vi "试验舱仿真器传递函数-带自然冷却10ms.vi"() -> ()   [LabVIEW 2018]
panel:
  out "波形图表":cluster{"上限":dbl, "上限":dbl, "上限":dbl}(graph)
  in  "自然冷却按钮":bool
  out "1.8m试验仓仓内温度":dbl(graph)
  out "1.8m试验仓仓内压力":dbl(graph)=-0.0229152
  out "1M8仓温度仿真":dbl(slide)=73.625 scale=0.0..250.0
  out "1M8仓压力仿真":dbl(slide)=-0.0229152 scale=0.0..1.0
  out "压力":dbl
  out "f 5":dbl format="%.3f"
  out "d排气影响压力":dbl
  out "f 4":dbl format="%.3f"
  out "d进蒸汽影响压力":dbl
  out "f 3":dbl format="%.3f"
  out "d进空气影响压力":dbl
  out "f 2":dbl format="%.3f"
  out "d进空气影响温度":dbl
  out "f":dbl format="%.3f"
  out "d进蒸汽影响温度":dbl
  out "温度":dbl
  # "试验舱"
  # "压力"
  # "温度"
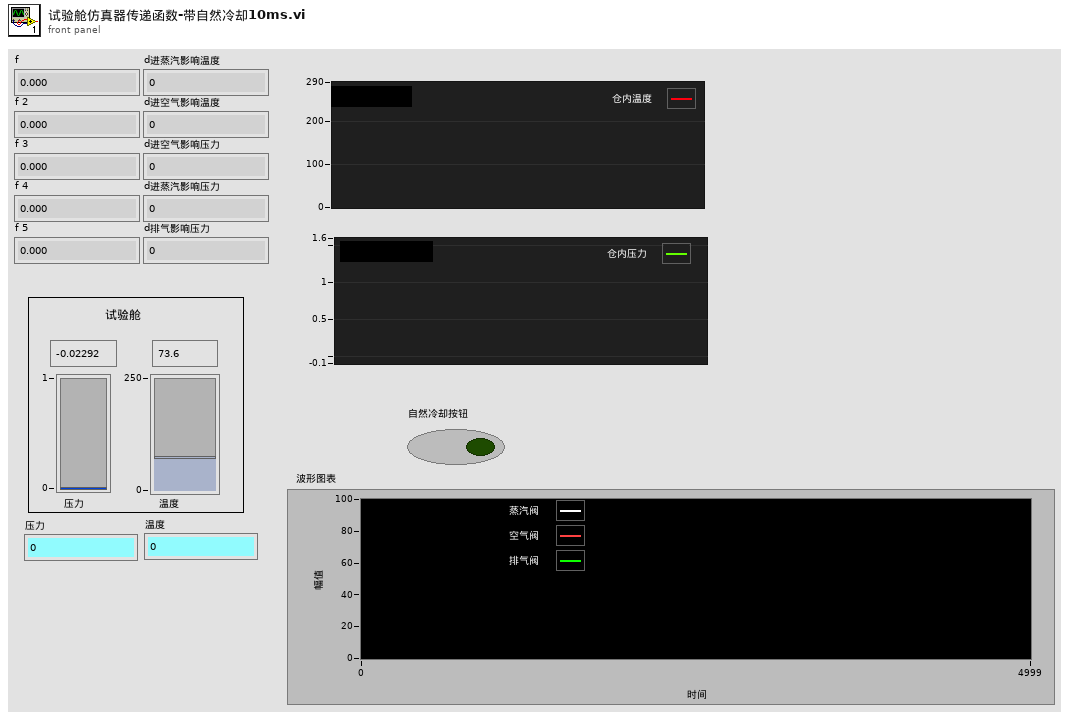
[diagram p1: front panel]
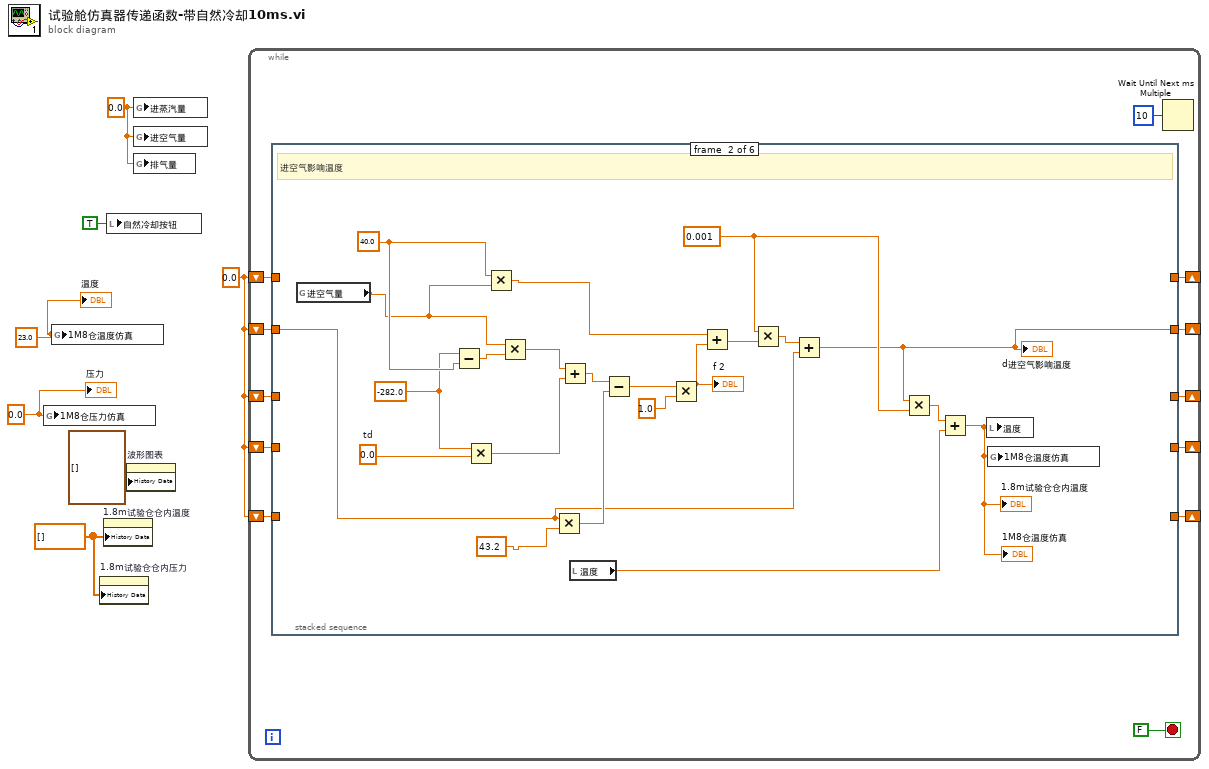
[diagram p0: block diagram]
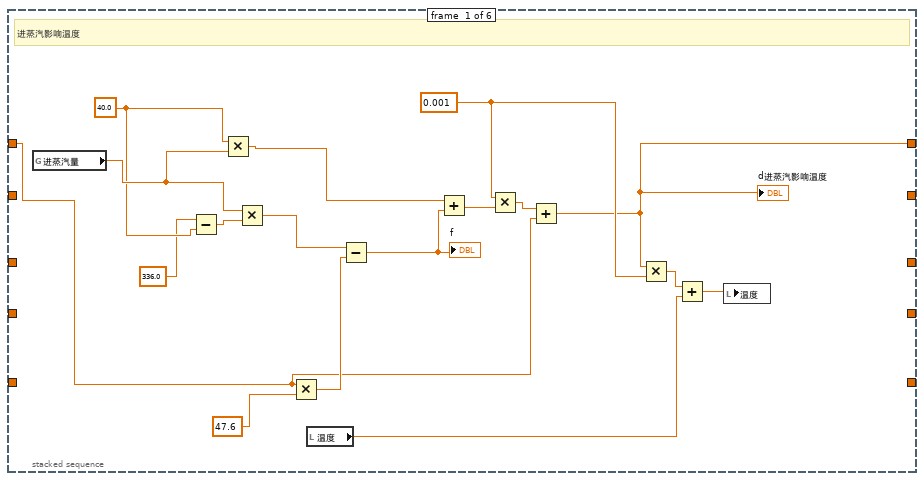
[diagram p2: hidden frame]
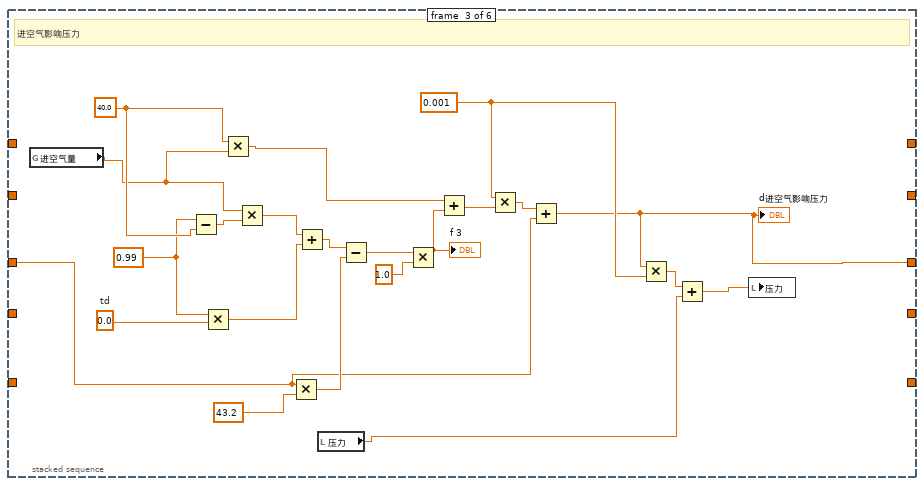
[diagram p3: hidden frame]
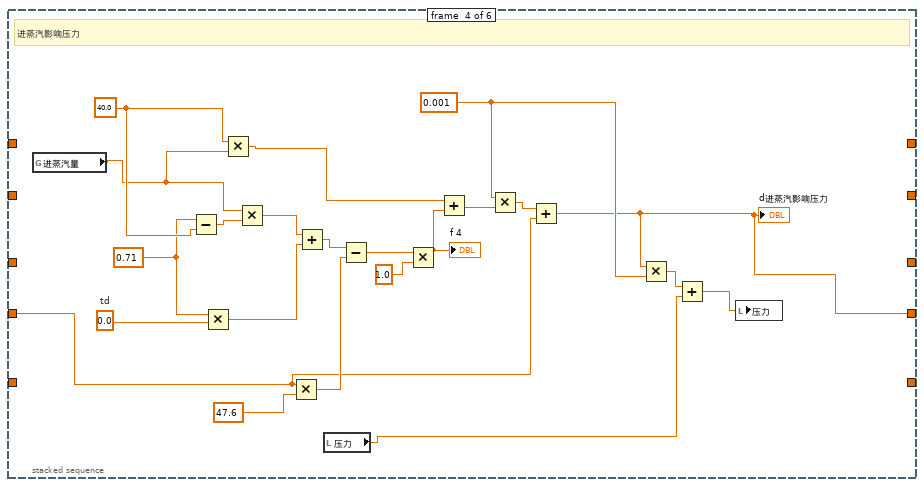
[diagram p4: hidden frame]
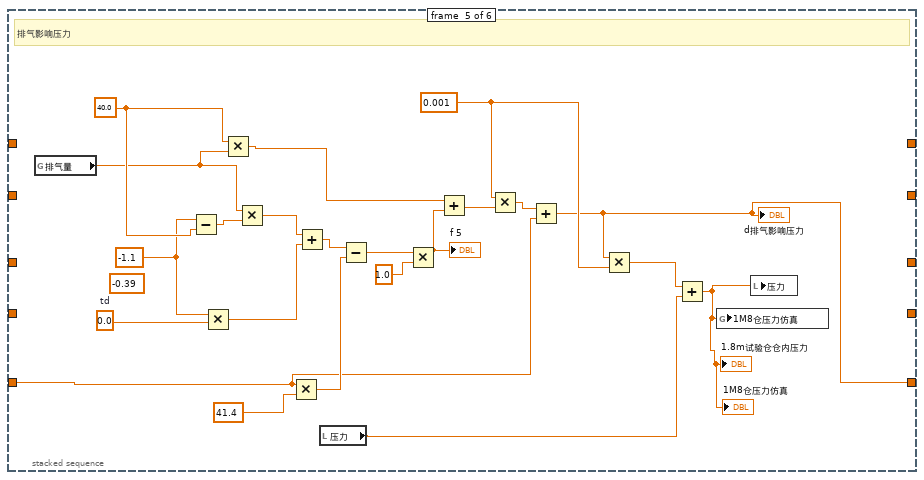
[diagram p5: hidden frame]
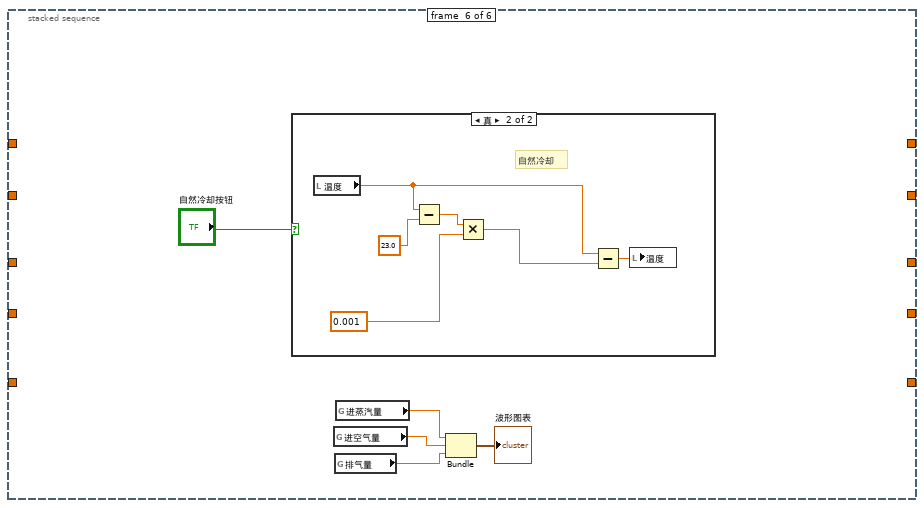
[diagram p6: hidden frame]
diagram:
  w3 = dbl[] [] ("历史数据")
  w6 = 0.0
  w7 = 0.0 ("进蒸汽量")
  w5 = 23.0 ("1.2m试验仓仓内温度")
  w4 = 0.0 ("1m2舱温度峰值")
  n1 = global write "全局变量.vi" "1M8仓压力仿真"(w4) -> ()
  n2 = global write "全局变量.vi" "1M8仓温度仿真"(w5) -> ()
  n3 = property on="1.8m试验仓仓内压力" class="WFChart (严格)"("History Data"=w3) -> ()  [unwired: 2 in, 2 out]
  n4 = property on="1.8m试验仓仓内温度" class="WFChart (严格)"("History Data"=w3) -> ()  [unwired: 2 in, 2 out]
  n5 = local write "自然冷却按钮"(TRUE ("自然冷却按钮")) -> ()
  n6 = property on="波形图表" class="WFChart (严格)"("History Data"=cluster{"上限":dbl, "上限":dbl, "上限":dbl}[] [] ("历史数据")) -> ()  [unwired: 2 in, 2 out]
  n7 = global write "全局变量.vi" "进蒸汽量"(w7) -> ()
  n8 = global write "全局变量.vi" "进空气量"(w7) -> ()
  n9 = global write "全局变量.vi" "排气量"(w7) -> ()
  n10 = while {
    shift-right: [w16] -> _
    shift-left: w6 -> [w17]
    shift-right: [w14] -> _
    shift-left: w6 -> [w15]
    shift-right: [w12] -> _
    shift-left: w6 -> [w13]
    shift-right: [w10] -> _
    shift-left: w6 -> [w11]
    shift-right: [w8] -> _
    shift-left: w6 -> [w9]
    stop <- FALSE stop-if-true
    n11 = stacked-sequence {
      tunnel: w17 -> [w24 _ _ _ _ _]
      tunnel: [w23 _ _ _ _ _] -> w16
      tunnel: w15 -> [_ w42 _ _ _ _]
      tunnel: [_ w41 _ _ _ _] -> w14
      tunnel: w13 -> [_ _ w65 _ _ _]
      tunnel: [_ _ w64 _ _ _] -> w12
      tunnel: w11 -> [_ _ _ w87 _ _]
      tunnel: [_ _ _ w86 _ _] -> w10
      tunnel: w9 -> [_ _ _ _ w109 _]
      tunnel: [_ _ _ _ w108 _] -> w8
      frame #0 {
        w34 = 40.0 ("b0")
        w33 = 0.001
        # "进蒸汽影响温度"
        n12 = global read "全局变量.vi" "进蒸汽量"() -> (w35:dbl)
        n13 = Subtract(x=336.0, y=w34) -> (x-y=w27:dbl)
        n14 = Multiply(x=w34, y=w35) -> (x*y=w26:dbl)
        n15 = Multiply(x=w35, y=w27) -> (x*y=w20:dbl)
        n16 = Multiply(x=w24, y=47.6) -> (x*y=w28:dbl)
        n17 = local read "温度"() -> (w36:dbl)
        n18 = Subtract(x=w20, y=w28) -> (x-y=w32:dbl)
        "f" <- w32
        n19 = Add(x=w26, y=w32) -> (x+y=w31:dbl)
        n20 = Multiply(x=w33, y=w31) -> (x*y=w30:dbl)
        n21 = Add(x=w30, y=w24) -> (x+y=w23:dbl)
        "d进蒸汽影响温度" <- w23
        n22 = Multiply(x=w23, y=w33) -> (x*y=w29:dbl)
        n23 = Add(x=w29, y=w36) -> (x+y=w25:dbl)
        n24 = local write "温度"(w25) -> ()
      }
      frame #1 {
        w57 = 0.0  # td
        w56 = 40.0 ("b0")
        w55 = 0.001
        w40 = -282.0 ("x")
        # "进空气影响温度"
        n25 = global read "全局变量.vi" "进空气量"() -> (w38:dbl)
        n26 = Subtract(x=w40, y=w56) -> (x-y=w44:dbl)
        n27 = Multiply(x=w40, y=w57) -> (x*y=w46:dbl)
        n28 = Multiply(x=w56, y=w38) -> (x*y=w43:dbl)
        n29 = Multiply(x=w38, y=w44) -> (x*y=w45:dbl)
        n30 = Multiply(x=w42, y=43.2) -> (x*y=w48:dbl)
        n31 = Add(x=w45, y=w46) -> (x+y=w47:dbl)
        n32 = local read "温度"() -> (w58:dbl)
        n33 = Subtract(x=w47, y=w48) -> (x-y=w49:dbl)
        n34 = Multiply(x=w49, y=1.0) -> (x*y=w53:dbl)
        "f 2" <- w53
        n35 = Add(x=w43, y=w53) -> (x+y=w52:dbl)
        n36 = Multiply(x=w55, y=w52) -> (x*y=w51:dbl)
        n37 = Add(x=w51, y=w42) -> (x+y=w41:dbl)
        "d进空气影响温度" <- w41
        n38 = Multiply(x=w41, y=w55) -> (x*y=w50:dbl)
        n39 = Add(x=w50, y=w58) -> (x+y=w37:dbl)
        "1.8m试验仓仓内温度" <- w37
        "1M8仓温度仿真" <- w37
        n40 = local write "温度"(w37) -> ()
        n41 = global write "全局变量.vi" "1M8仓温度仿真"(w37) -> ()
      }
      frame #2 {
        w80 = 0.0  # td
        w79 = 40.0 ("b0")
        w78 = 0.001
        w63 = 0.99 ("x")
        # "进空气影响压力"
        n42 = global read "全局变量.vi" "进空气量"() -> (w61:dbl)
        n43 = Subtract(x=w63, y=w79) -> (x-y=w67:dbl)
        n44 = Multiply(x=w63, y=w80) -> (x*y=w69:dbl)
        n45 = Multiply(x=w79, y=w61) -> (x*y=w66:dbl)
        n46 = Multiply(x=w61, y=w67) -> (x*y=w68:dbl)
        n47 = Multiply(x=w65, y=43.2) -> (x*y=w71:dbl)
        n48 = Add(x=w68, y=w69) -> (x+y=w70:dbl)
        n49 = local read "压力"() -> (w60:dbl)
        n50 = Subtract(x=w70, y=w71) -> (x-y=w72:dbl)
        n51 = Multiply(x=w72, y=1.0) -> (x*y=w76:dbl)
        "f 3" <- w76
        n52 = Add(x=w66, y=w76) -> (x+y=w75:dbl)
        n53 = Multiply(x=w78, y=w75) -> (x*y=w74:dbl)
        n54 = Add(x=w74, y=w65) -> (x+y=w64:dbl)
        "d进空气影响压力" <- w64
        n55 = Multiply(x=w64, y=w78) -> (x*y=w73:dbl)
        n56 = Add(x=w73, y=w60) -> (x+y=w59:dbl)
        n57 = local write "压力"(w59) -> ()
      }
      frame #3 {
        w102 = 0.0  # td
        w101 = 40.0 ("b0")
        w100 = 0.001
        w85 = 0.71 ("x")
        # "进蒸汽影响压力"
        n58 = global read "全局变量.vi" "进蒸汽量"() -> (w83:dbl)
        n59 = Subtract(x=w85, y=w101) -> (x-y=w89:dbl)
        n60 = Multiply(x=w85, y=w102) -> (x*y=w91:dbl)
        n61 = Multiply(x=w101, y=w83) -> (x*y=w88:dbl)
        n62 = Multiply(x=w83, y=w89) -> (x*y=w90:dbl)
        n63 = Multiply(x=w87, y=47.6) -> (x*y=w93:dbl)
        n64 = Add(x=w90, y=w91) -> (x+y=w92:dbl)
        n65 = local read "压力"() -> (w82:dbl)
        n66 = Subtract(x=w92, y=w93) -> (x-y=w94:dbl)
        n67 = Multiply(x=w94, y=1.0) -> (x*y=w98:dbl)
        "f 4" <- w98
        n68 = Add(x=w88, y=w98) -> (x+y=w97:dbl)
        n69 = Multiply(x=w100, y=w97) -> (x*y=w96:dbl)
        n70 = Add(x=w96, y=w87) -> (x+y=w86:dbl)
        "d进蒸汽影响压力" <- w86
        n71 = Multiply(x=w86, y=w100) -> (x*y=w95:dbl)
        n72 = Add(x=w95, y=w82) -> (x+y=w81:dbl)
        n73 = local write "压力"(w81) -> ()
      }
      frame #4 {
        (unwired) -0.39 ("x")
        w124 = 0.0  # td
        w123 = 40.0 ("b0")
        w122 = 0.001
        w107 = -1.1 ("x")
        # "排气影响压力"
        n74 = global read "全局变量.vi" "排气量"() -> (w105:dbl)
        n75 = Subtract(x=w107, y=w123) -> (x-y=w111:dbl)
        n76 = Multiply(x=w107, y=w124) -> (x*y=w113:dbl)
        n77 = Multiply(x=w123, y=w105) -> (x*y=w110:dbl)
        n78 = Multiply(x=w105, y=w111) -> (x*y=w112:dbl)
        n79 = Multiply(x=w109, y=41.4) -> (x*y=w115:dbl)
        n80 = Add(x=w112, y=w113) -> (x+y=w114:dbl)
        n81 = local read "压力"() -> (w104:dbl)
        n82 = Subtract(x=w114, y=w115) -> (x-y=w116:dbl)
        n83 = Multiply(x=w116, y=1.0) -> (x*y=w120:dbl)
        "f 5" <- w120
        n84 = Add(x=w110, y=w120) -> (x+y=w119:dbl)
        n85 = Multiply(x=w122, y=w119) -> (x*y=w118:dbl)
        n86 = Add(x=w118, y=w109) -> (x+y=w108:dbl)
        "d排气影响压力" <- w108
        n87 = Multiply(x=w108, y=w122) -> (x*y=w117:dbl)
        n88 = Add(x=w117, y=w104) -> (x+y=w103:dbl)
        "1M8仓压力仿真" <- w103
        "1.8m试验仓仓内压力" <- w103
        n89 = global write "全局变量.vi" "1M8仓压力仿真"(w103) -> ()
        n90 = local write "压力"(w103) -> ()
      }
      frame #5 {
        n91 = case shown="真" "自然冷却按钮" {
          frame False {
          }
          frame True {
            # "自然冷却"
            n92 = local read "温度"() -> (w134:dbl)
            n93 = Subtract(x=w134, y=23.0) -> (x-y=w132:dbl)
            n94 = Multiply(x=w132, y=0.001) -> (x*y=w130:dbl)
            n95 = Subtract(x=w134, y=w130) -> (x-y=w135:dbl)
            n96 = local write "温度"(w135) -> ()
          }
        }
        n97 = global read "全局变量.vi" "进空气量"() -> (w126:dbl)
        n98 = global read "全局变量.vi" "排气量"() -> (w125:dbl)
        n99 = global read "全局变量.vi" "进蒸汽量"() -> (w127:dbl)
        n100 = Bundle("进蒸汽量"=w127, "进空气量"=w126, "排气量"=w125) -> (→"波形图表":cluster{"进蒸汽量":dbl, "进空气量":dbl, "排气量":dbl})  [unwired: 1 in]
      }
    }
    n101 = Wait Until Next ms Multiple(millisecond multiple=u32 10) -> ()  [unwired: 1 out]
  }
  "温度" <- w5
  "压力" <- w4
